vi "Drive Modifications.vi"(1 "Drive Global Data In":T1) -> (0 "Drive Global Data Out":T1)   [LabVIEW 2013]
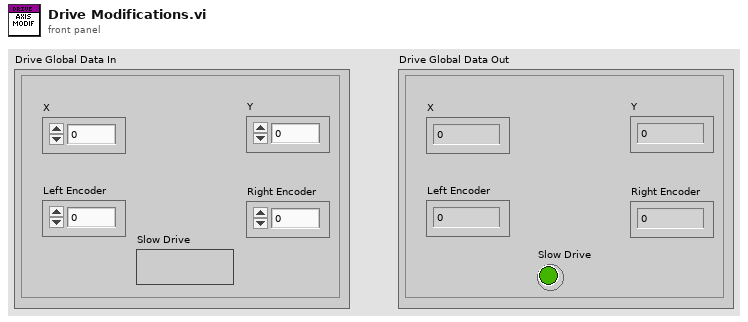
[diagram p1: front panel]
types:
  T1 = cluster{"Y":dbl, "X":dbl, "Left Encoder":dbl, "Right Encoder":dbl, "Slow Drive":bool}
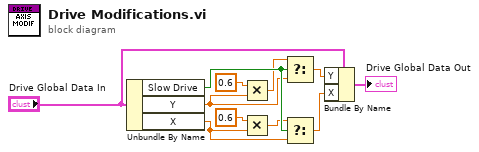
[diagram p0: block diagram]
diagram:
  n1 = Unbundle By Name("Drive Global Data In") -> ("Slow Drive"=w9:bool, "Y"=w7:dbl, "X"=w4:dbl)
  n2 = Multiply(x=0.6 ("t"), y=w7) -> (x*y=w6:dbl)
  n3 = Multiply(x=0.6 ("t"), y=w4) -> (x*y=w3:dbl)
  n4 = Select(t=w6, s=w9, f=w7) -> (s? t:f=w1:dbl)
  n5 = Select(t=w3, s=w9, f=w4) -> (s? t:f=w2:dbl)
  n6 = Bundle By Name(cluster="Drive Global Data In", "Y"=w1, "X"=w2) -> (→"Drive Global Data Out":T1)
